vi "Shake preStep.vi"(8 "error in (no error)":errorcluster, 11 "TapeDrive in":refnum<class "TapeDrive.lvclass">) -> (0 "error out":errorcluster, 3 "TapeDrive out":refnum<class "TapeDrive.lvclass">)   [LabVIEW 2020, in "TapeDrive.lvclass"]
uses:
  TapeDrive.lvclass
  TapeDrive.lvclass/TapeDrive.ctl
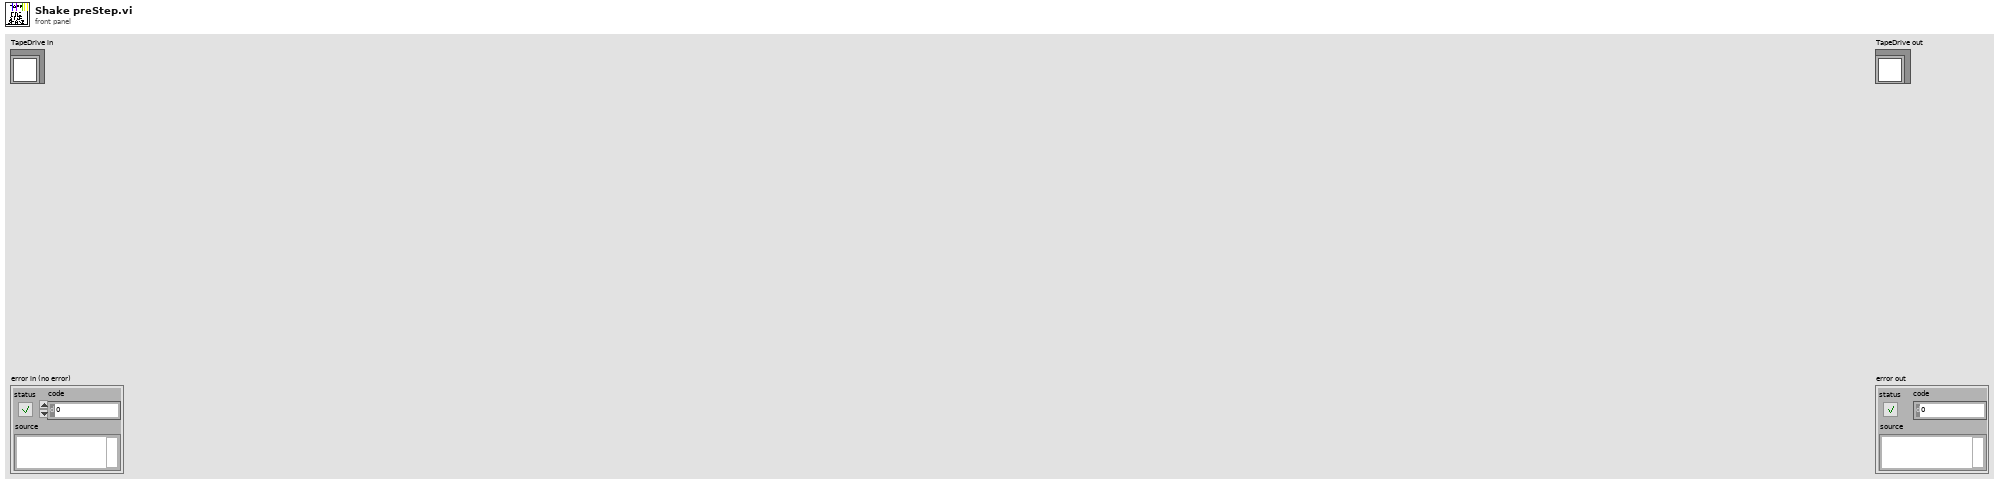
[diagram p1: front panel]
types:
  T1 = typedef "OnOffTypeDef.ctl" = enum16{"off", "on"}
  T2 = typedef "Direction_TypDef.ctl" = enum16{"left", "right"}
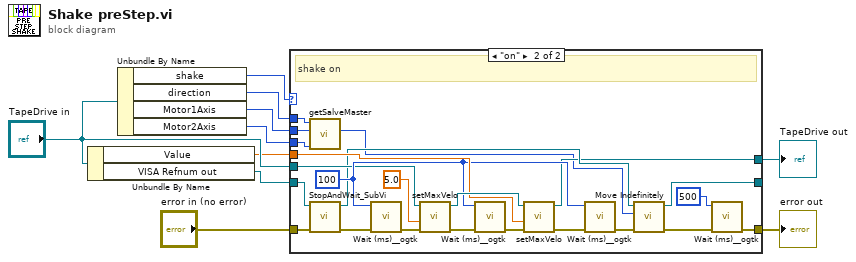
[diagram p0: block diagram]
diagram:
  n1 = Unbundle By Name("TapeDrive in") -> ("Value"=w4:dbl, "VISA Refnum out"=w3:refnum<visa-resource-name>)
  n2 = Unbundle By Name("TapeDrive in") -> ("shake"=w6:T1, "direction"=w8:T2, "Motor1Axis"=w9:i32, "Motor2Axis"=w10:i32)
  n3 = case shown="\"on\"" w6 {
    tunnel: w3 -> [w13 w36]
    tunnel: [w13 w35] -> _
    tunnel: "error in (no error)" -> [w12 w34]
    tunnel: [w12 w23] -> w2
    tunnel: w4 -> [_ w25]
    tunnel: "TapeDrive in" -> [w11 w20]
    tunnel: [w11 w18] -> w5
    tunnel: w8 -> [_ w17]
    tunnel: w9 -> [_ w16]
    tunnel: w10 -> [_ w15]
    frame "off", Default {
    }
    frame "on" {
      w22 = u32 100 ("milliseconds to wait")
      # "shake on"
      n4 = call "getSalveMaster.vi"("Motor2Axis"=w15, "Motor1Axis"=w16, "direction"=w17) -> ("Master"=w14:i32)  [unwired: 7 in, 1 out]
      n5 = call "StopAndWait_SubVi.vi"("error in (no error)"=w34, "VISA Refnum in"=w36) -> ("error out"=w33:errorcluster, "VISA Refnum out"=w19:refnum<visa-resource-name>)  [unwired: 8 in]
      n6 = call <userlib>:"Wait (ms)__ogtk.vi"("error in (no error)"=w33, "milliseconds to wait"=w22) -> ("error out"=w32:errorcluster)  [unwired: 8 in, 1 out]
      n7 = call "setMaxVelo.vi"("error in (no error)"=w32, "NewVal"=5.0, "TapeDrive in"=w20) -> ("error out"=w30:errorcluster, "TapeDrive out"=w26:refnum<class "TapeDrive.lvclass">)  [unwired: 6 in, 1 out]
      n8 = call <userlib>:"Wait (ms)__ogtk.vi"("error in (no error)"=w30, "milliseconds to wait"=w22) -> ("error out"=w29:errorcluster)  [unwired: 8 in, 1 out]
      n9 = call "setMaxVelo.vi"("error in (no error)"=w29, "NewVal"=w25, "TapeDrive in"=w26) -> ("error out"=w28:errorcluster, "TapeDrive out"=w18:refnum<class "TapeDrive.lvclass">)  [unwired: 6 in, 1 out]
      n10 = call <userlib>:"Wait (ms)__ogtk.vi"("error in (no error)"=w28, "milliseconds to wait"=w22) -> ("error out"=w27:errorcluster)  [unwired: 8 in, 1 out]
      n11 = call "Move Indefinitely.vi"("error in (no error)"=w27, "Axis (1)"=w14, "VISA resource name"=w19) -> ("error out"=w24:errorcluster, "VISA resource name out"=w35:refnum<visa-resource-name>)  [unwired: 3 in]
      n12 = call <userlib>:"Wait (ms)__ogtk.vi"("error in (no error)"=w24, "milliseconds to wait"=u32 500) -> ("error out"=w23:errorcluster)  [unwired: 8 in, 1 out]
    }
  }
  "TapeDrive out" <- w5
  "error out" <- w2
